vi "Parameter Set.vi"(8 "error in (no error)":errorcluster, 11 "Power Meter in":refnum<class "Power Meter.lvclass">) -> (0 "error out":errorcluster, 3 "Power Meter out":refnum<class "Power Meter.lvclass">)   [LabVIEW 2009, in "Power Meter.lvclass"]
doc: "Opens pop-up window for changing Newport 1830-C parameter settings within another control panel."
uses:
  Power Meter.lvclass
  Power Meter.lvclass/Power Meter.ctl
panel:
  out "Error":bool
  in  "stop":bool
  in  "R2C":bool
  in  "Averaging Time":dbl[unit]=0.5
  in  "Averaging?":bool
  in  "Local Lockout (0:1)":u32(ring) items=["Off", "On"]
  in  "ATTN (0:1)":u32(ring)=1 items=["Off", "On"]
  in  "Run/Stop (1:0)":u32(ring)=1 items=["Stop", "Run"]
  in  "AVG (1:3)":u32(ring)=2 items=["Slow"=1, "Medium"=2, "Fast"=3]
  in  "Units (1:4)":u32(ring)=1 items=["W"=1, "dB"=2, "dBm"=3, "REL"=4]
  in  "Zero (0:1)":u32(ring) items=["Off", "On"]
  in  "Beeper (0:1)":u32(ring) items=["Off", "On"]
  in  "Backlight (0:2)":u32(ring)=1 items=["Off", "Low", "High"]
  in  "Range (0-Auto,1:8)":u32(ring) items=["Auto", "Lowest", "2", "3", "4", "5", "6", "7", "Highest"]
  in  "Wavelength (nnnn)":dbl[unit]=8.210000000000001e-07
  in  "Set":bool
  # "Only use Watts with LPC!"
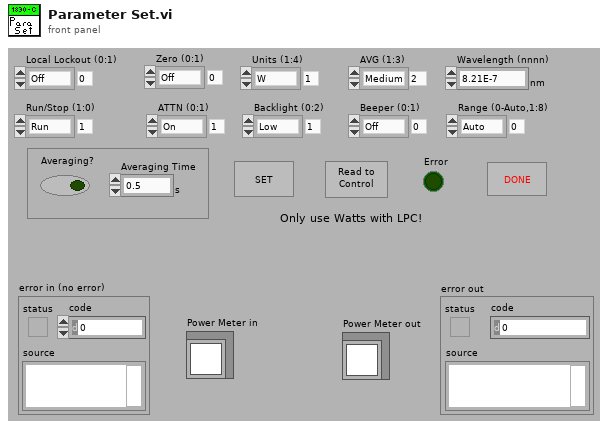
[diagram p1: front panel]
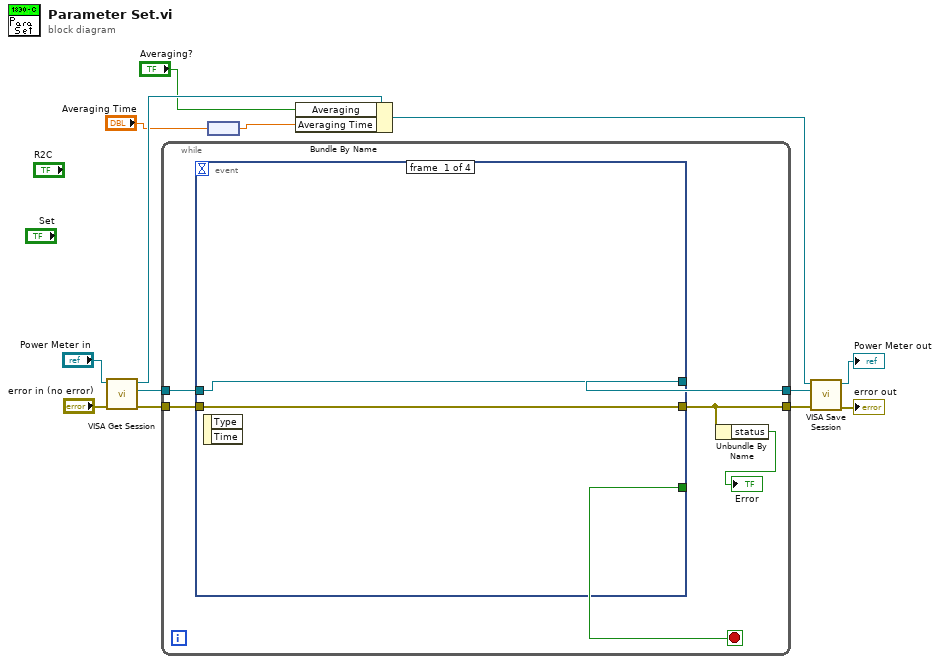
[diagram p0: block diagram]
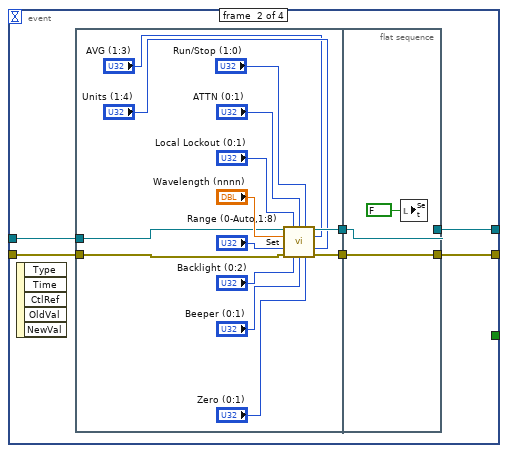
[diagram p2: hidden frame]
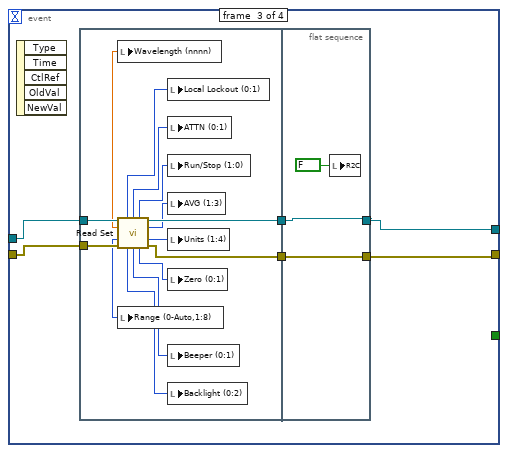
[diagram p3: hidden frame]
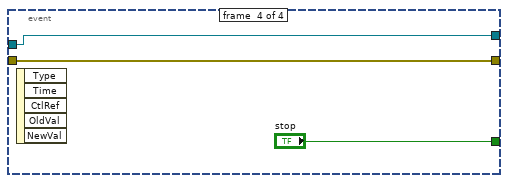
[diagram p4: hidden frame]
diagram:
  n1 = call-dynamic "VISA Get Session.vi"("error in (no error)"="error in (no error)", "Instrument.lvclass in"="Power Meter in") -> ("error out"=w13:errorcluster, "VISA Resource Name"=w12:refnum<visa-resource-name>, "Instrument.lvclass out"=w5:refnum<class "Power Meter.lvclass">)  [unwired: 6 in, 1 out]
  n2 = while {
    tunnel: w13 -> [w19]
    tunnel: w12 -> [w18]
    tunnel: [w17] -> w10
    tunnel: [w15] -> w9
    stop <- w16 stop-if-true
    n3 = event shown="[1] \"Set\": Value Change" {
      selector: _ -> [_ _ _ _]
      dyn-events: _ -> [_ _ _ _]
      timeout: _ -> [_ _ _ _]
      tunnel: [w21 w27 w49 w70] -> w17
      tunnel: w19 -> [w20 w26 w48 w69]
      tunnel: [w20 w25 w47 w69] -> w15
      tunnel: w18 -> [w21 w24 w50 w70]
      tunnel: [_ _ _ "stop"] -> w16
      event #0 {
        n4 = event-data() -> ()  [unwired: 1 in, 2 out]
      }
      event #1 {
        n5 = event-data() -> ()  [unwired: 1 in, 5 out]
        n6 = flat-sequence {
          tunnel: [w41] -> w23
          tunnel: w26 -> [w38]
          tunnel: [w34] -> w22
          tunnel: w24 -> [w28]
          tunnel: [w43] -> w27
          tunnel: w23 -> [w43]
          tunnel: [w42] -> w25
          tunnel: w22 -> [w42]
          frame #0 {
            n7 = call "Set.vi"("VISA resource name"=w28, "Local Lockout (0:1)"="Local Lockout (0:1)", "ATTN (0:1)"="ATTN (0:1)", "Run/Stop (1:0)"="Run/Stop (1:0)", "Wavelength (nnnn)"="Wavelength (nnnn)", "AVG (1:3)"="AVG (1:3)", "Range (0-Auto,1:8)"="Range (0-Auto,1:8)", "Units (1:4)"="Units (1:4)", "error in (no error)"=w38, "Backlight (0:2)"="Backlight (0:2)", "Beeper (0:1)"="Beeper (0:1)", "Zero (0:1)"="Zero (0:1)") -> ("VISA resource name out"=w41:refnum<visa-resource-name>, "error out"=w34:errorcluster)  [unwired: 2 in]
          }
          frame #1 {
            n8 = local write "Set"(FALSE ("Set")) -> ()
          }
        }
      }
      event #2 {
        n9 = event-data() -> ()  [unwired: 1 in, 5 out]
        n10 = flat-sequence {
          tunnel: w50 -> [w64]
          tunnel: [w63] -> w46
          tunnel: w48 -> [w62]
          tunnel: [w61] -> w45
          tunnel: [w66] -> w49
          tunnel: w46 -> [w66]
          tunnel: [w65] -> w47
          tunnel: w45 -> [w65]
          frame #0 {
            n11 = call "Read Set.vi"("VISA resource name"=w64, "error in (no error)"=w62) -> ("Local Lockout"=w60:u32, "ATTN"=w59:u32, "Run/Stop"=w58:u32, "VISA resource name out"=w63:refnum<visa-resource-name>, "Wavelength (nnnn)"=w52:dbl[unit], "AVG"=w57:u32, "Range (1:8)"=w51:u32, "Units"=w56:u32, "Backlight"=w55:u32, "Beeper"=w54:u32, "Zero"=w53:u32, "error out"=w61:errorcluster)  [unwired: 2 in]
            n12 = local write "Wavelength (nnnn)"(w52) -> ()
            n13 = local write "Range (0-Auto,1:8)"(w51) -> ()
            n14 = local write "Local Lockout (0:1)"(w60) -> ()
            n15 = local write "ATTN (0:1)"(w59) -> ()
            n16 = local write "Run/Stop (1:0)"(w58) -> ()
            n17 = local write "AVG (1:3)"(w57) -> ()
            n18 = local write "Units (1:4)"(w56) -> ()
            n19 = local write "Zero (0:1)"(w53) -> ()
            n20 = local write "Beeper (0:1)"(w54) -> ()
            n21 = local write "Backlight (0:2)"(w55) -> ()
          }
          frame #1 {
            n22 = local write "R2C"(FALSE ("R2C")) -> ()
          }
        }
      }
      event #3 {
        n23 = event-data() -> ()  [unwired: 1 in, 5 out]
      }
    }
    n24 = Unbundle By Name(w15) -> ("status"=→"Error":bool)
  }
  n25 = node("Averaging Time") -> (w2:dbl)
  n26 = Bundle By Name(cluster=w5, "Averaging"="Averaging?", "Averaging Time"=w2) -> (w1:refnum<class "Power Meter.lvclass">)
  n27 = call-dynamic "VISA Save Session.vi"("error in (no error)"=w9, "VISA Resource Name"=w10, "Instrument.lvclass in"=w1) -> ("error out"=→"error out":errorcluster, "Instrument.lvclass out"=→"Power Meter out":refnum<class "Power Meter.lvclass">)  [unwired: 7 in]
